vi "Add Wrapper to Library - Multiple Converter.vi"(11 "error in":errorcluster) -> (15 "error out":errorcluster)   [LabVIEW 2021, in "Converter.lvlib"]
uses:
  Converter.lvlib
  Path Functions/Path Functions.lvlib
  Converter Reusables/Converter Reusables.lvlib
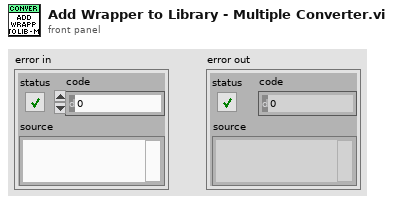
[diagram p1: front panel]
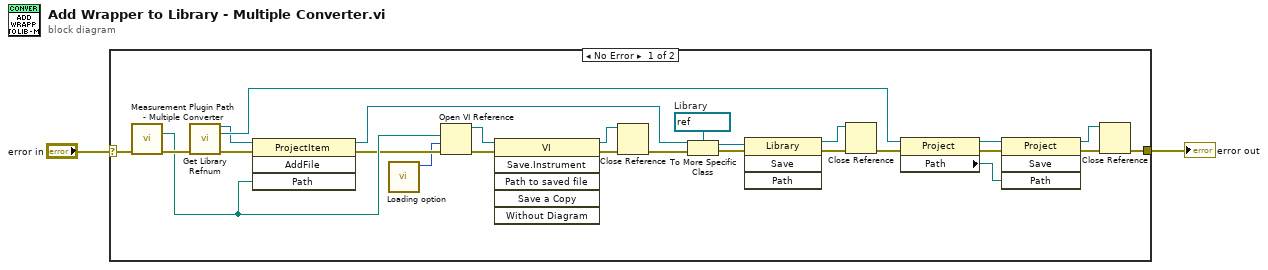
[diagram p0: block diagram]
diagram:
  n1 = case shown="No Error" "error in" {
    selector: "error in" -> [w19 w29]
    tunnel: [w26 w29] -> w2
    frame No Error {
      w15 = refnum<vi> refnum  # Library
      n2 = call "Measurement Plugin Path - Multiple Converter.vi"("error in"=w19) -> ("wrapper path"=w8:path, "error out"=w18:errorcluster)  [unwired: 2 in, 11 out]
      n3 = call "Get Library Refnum.vi"("error in"=w18) -> ("library refnum"=w16:refnum<vi>, "project refnum"=w24:refnum<vi>, "error out"=w20:errorcluster)  [unwired: 12 in]
      n4 = invoke class="ProjectItem" method="AddFile"(reference=w16, error in=w20, "Path"=w8) -> (reference out=w12:refnum<vi>, error out=w6:errorcluster)  [unwired: 1 in, 2 out]
      n5 = call "Loading option.vi"() -> ("options"=w3:i32)  [unwired: 11 in]
      n6 = Open VI Reference(vi path=w8, options=w3, error in (no error)=w6) -> (vi reference=w7:refnum<vi>, error out=w5:errorcluster)  [unwired: 3 in]
      n7 = invoke class="VI" method="Save.Instrument"(reference=w7, error in=w5) -> (reference out=w9:refnum<vi>, error out=w10:errorcluster)  [unwired: 4 in, 4 out]
      n8 = Close Reference(reference=w9, error in (no error)=w10) -> (error out=w17:errorcluster)
      n9 = To More Specific Class(target class=w15, reference=w12, error in=w17) -> (specific class reference=w14:refnum<vi>, error out=w13:errorcluster)
      n10 = invoke class="Library" method="Save"(reference=w14, error in=w13) -> (reference out=w23:refnum<vi>, error out=w22:errorcluster)  [unwired: 2 in, 2 out]
      n11 = Close Reference(reference=w23, error in (no error)=w22) -> (error out=w21:errorcluster)
      n12 = property class="Project"(reference=w24, error in=w21) -> (reference out=w11:refnum<vi>, error out=w27:errorcluster, "Path"=w4:path)
      n13 = invoke class="Project" method="Save"(reference=w11, error in=w27, "Path"=w4) -> (reference out=w25:refnum<vi>, error out=w28:errorcluster)  [unwired: 1 in, 2 out]
      n14 = Close Reference(reference=w25, error in (no error)=w28) -> (error out=w26:errorcluster)
    }
    frame Error {
    }
  }
  "error out" <- w2
